vi "MAG PREP.vi"(0 "VISA In":refnum<visa-resource-name>, 5 "MagQ":refnum<queue>, 7 "Boolean":bool, 9 "PSU Status In":T1 {"Trip Current" format="%.3f"; "Trip Field" format="%.4f"; "Voltage" format="%.2f"; "Field Constant" format="%.6f"; "MID Setpoint (T)" format="%.4f"; "MID Setpoint (A)" format="%.3f"; "MAX Setpoint (T)" format="%.4f"; "MAX Setpoint (A)" format="%.3f"; "Heater Voltage" format="%.2f"; "V Limit (V)" format="%.2f"; "Ramp Rate (A/s)" format="%.3f"; "Output (A)" format="%.3f"; "Output (T)" format="%.4f"; "Persistent Current" format="%.3f"; "Persistent Field" format="%.4f"}, 11 "Error In":errorcluster) -> (4 "VISA Out":refnum<visa-resource-name>, 6 "MagQ":refnum<queue>, 10 "PSU Status Out":T1 {"Trip Current" format="%.3f"; "Trip Field" format="%.4f"; "Voltage" format="%.2f"; "Field Constant" format="%.6f"; "MID Setpoint (T)" format="%.4f"; "MID Setpoint (A)" format="%.3f"; "MAX Setpoint (T)" format="%.4f"; "MAX Setpoint (A)" format="%.3f"; "Heater Voltage" format="%.2f"; "V Limit (V)" format="%.2f"; "Ramp Rate (A/s)" format="%.3f"; "Output (A)" format="%.3f"; "Output (T)" format="%.4f"; "Persistent Current" format="%.3f"; "Persistent Field" format="%.4f"}, 15 "error out":errorcluster)   [LabVIEW 2025]
uses:
  <instrlib>/SMS LabVIEW Drivers/Source Code/Cryogenic Ltd SMSXXX.lvlib
  <instrlib>/SMS LabVIEW Drivers/Source Code/Public/PSU Status.ctl
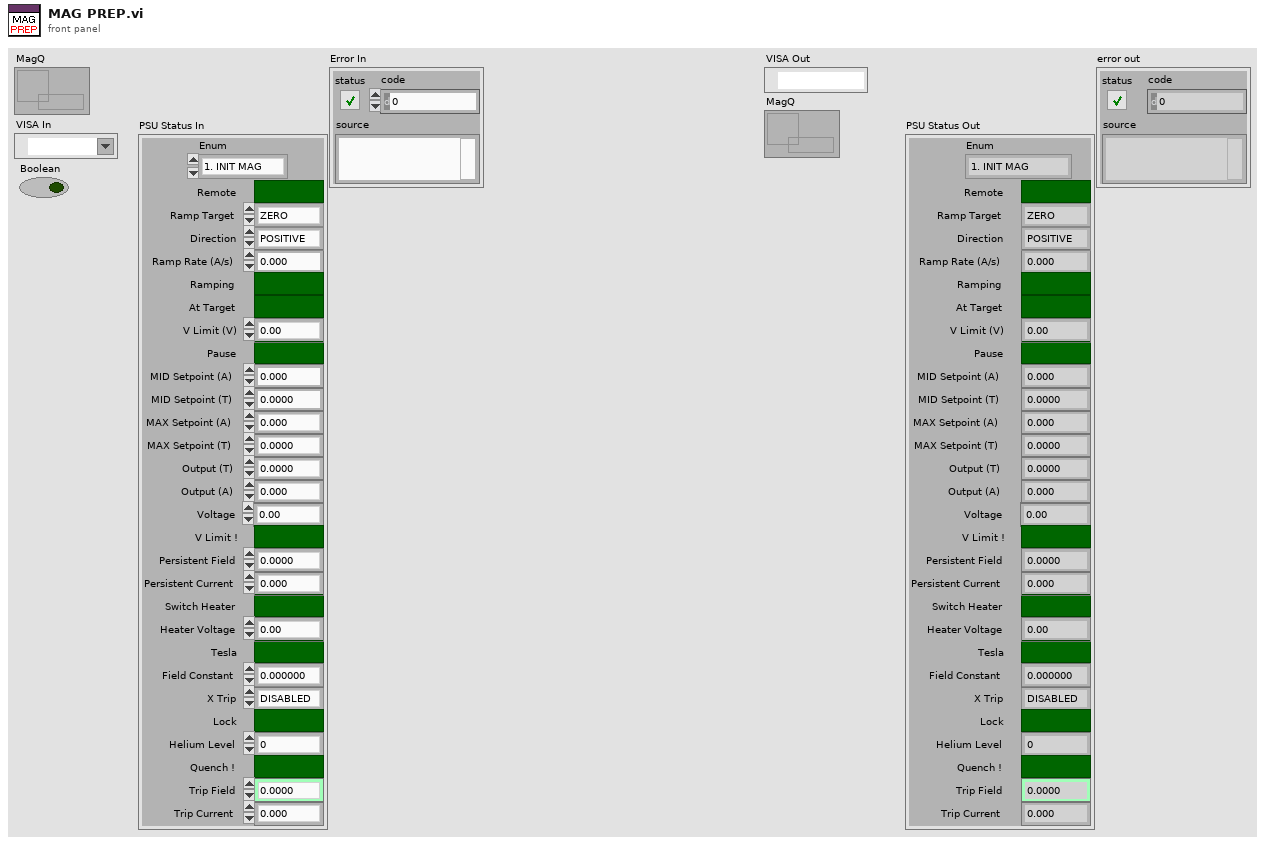
[diagram p1: front panel]
types:
  T1 = typedef "Cryogenic Ltd SMSXXX.lvlib/PSU Status.ctl" = cluster{"Ramp Target":enum16{"ZERO", "MID", "MAX"}, "Pause":bool, "Switch Heater":bool, "Persistent Field":dbl, "Persistent Current":dbl, "Tesla":bool, "Output (T)":dbl, "Output (A)":dbl, "X Trip":enum16{"DISABLED", "ENABLED", "ACTIVE"}, "Ramp Rate (A/s)":dbl, "V Limit (V)":dbl, "Heater Voltage":dbl, "MAX Setpoint (A)":dbl, "MAX Setpoint (T)":dbl, "MID Setpoint (A)":dbl, "MID Setpoint (T)":dbl, "Lock":bool, "Field Constant":dbl, "Remote":bool, "Direction":enum16{"POSITIVE", "NEGATIVE", "OPEN", "UNIPOLAR"}, "Helium Level":u16, "Quench !":bool, "Voltage":dbl, "V Limit !":bool, "Ramping":bool, "At Target":bool, "Trip Field":dbl, "Trip Current":dbl, "Enum":enum16{"1. INIT MAG", "2. MAG ON ", "3. MAG_STAB", "4. MAG IDLE", "5. NEXT FIELD", "6. MAG OFF (Reset)"}}
  T2 = enum16{"1. INIT MAG", "2. MAG ON", "3. MAG_STAB", "4. MAG IDLE", "5. PREP NEXT FIELD", "6. APPLY NEXT FIELD", "7. PREP OFF", "8. MAG OFF (Reset)"}
  T3 = enum16{"RAMP TO ZERO", "RAMP TO MID", "RAMP TO MAX"}
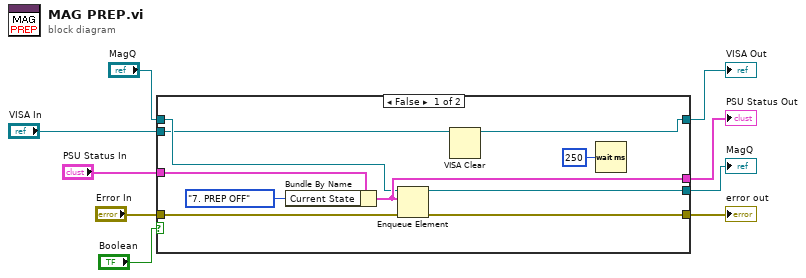
[diagram p0: block diagram]
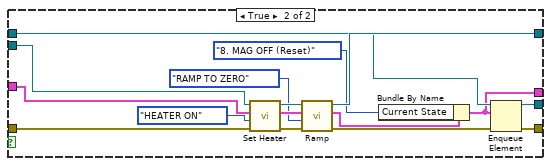
[diagram p2: hidden frame]
diagram:
  n1 = case shown="False" "Boolean" {
    tunnel: "Error In" -> [w17 w28]
    tunnel: "VISA In" -> [w13 w30]
    tunnel: "PSU Status In" -> [w16 w29]
    tunnel: [w12 w27] -> w4
    tunnel: [w15 w24] -> w3
    tunnel: [w18 w22] -> w1
    tunnel: [w19 w21] -> w2
    tunnel: "MagQ" -> [w14 w26]
    frame False {
      n2 = Bundle By Name(cluster=w16, "Current State"=T2."7. PREP OFF") -> (w15:T1)
      n3 = Enqueue Element(queue=w14, element=w15, error in (no error)=w17) -> (queue out=w19:refnum<queue>, error out=w18:errorcluster)  [unwired: 1 in, 1 out]
      n4 = VISA Clear(VISA resource name=w13) -> (VISA resource name out=w12:refnum<visa-resource-name>)  [unwired: 1 in, 1 out]
      n5 = Wait (ms)(milliseconds to wait=u32 250) -> ()  [unwired: 1 out]
    }
    frame True {
      n6 = call <instrlib>:"Set Heater.vi"("Error in (no error)"=w28, "Heater (On/Off)"=enum16{"HEATER OFF", "HEATER ON"}."HEATER ON", "PSU Status In"=w29, "VISA Resource Name In"=w30) -> ("Error out"=w32:errorcluster, "PSU Status Out"=w33:T1, "VISA Resource Name Out"=w34:refnum<visa-resource-name>)  [unwired: 4 in, 1 out]
      n7 = call <instrlib>:"Ramp.vi"("Error in (no error)"=w32, "Ramp Target"=T3."RAMP TO ZERO", "PSU Status In"=w33, "VISA Resource Name In"=w34) -> ("Error out"=w23:errorcluster, "PSU Status Out"=w25:T1, "VISA Resource Name Out"=w27:refnum<visa-resource-name>)  [unwired: 4 in, 1 out]
      n8 = Bundle By Name(cluster=w25, "Current State"=T2."8. MAG OFF (Reset)") -> (w24:T1)
      n9 = Enqueue Element(queue=w26, element=w24, error in (no error)=w23) -> (queue out=w21:refnum<queue>, error out=w22:errorcluster)  [unwired: 1 in, 1 out]
    }
  }
  "VISA Out" <- w4
  "PSU Status Out" <- w3
  "MagQ" <- w2
  "error out" <- w1
